vi "argosclient.vi"() -> ()   [LabVIEW 2014]
panel:
  out "locking":string
  in  "stop":bool
  out "bscale":dbl format="%#_9g"
  in  "set locking":bool
  in  "wnum setpoint":dbl=2284.249 format="%#_13g"
  in  "bscale":dbl=1.0 min=0.0001 max=1.0 step=0.0001 format="%#_13g"
  in  "locking":enum16{"off", "reg a", "reg b"}(ring)
  out "wnum measured":dbl format="%#_9g"
  in  "set bscale":bool
  in  "set wnum":bool
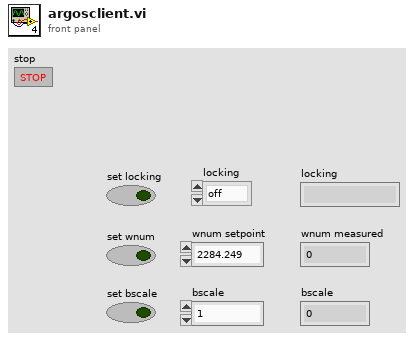
[diagram p1: front panel]
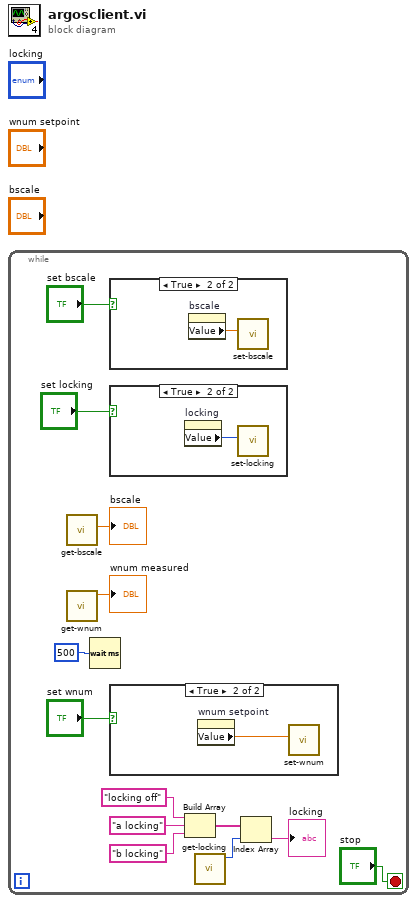
[diagram p0: block diagram]
diagram:
  n1 = while {
    stop <- "stop" stop-if-true
    n2 = call "get-bscale.vi"() -> ("bscale"=→"bscale":dbl)  [unwired: 10 in, 1 out]
    n3 = call "get-wnum.vi"() -> ("wnum"=→"wnum measured":dbl)  [unwired: 10 in, 1 out]
    n4 = Wait (ms)(milliseconds to wait=u32 500) -> ()  [unwired: 1 out]
    n5 = case shown="True" "set bscale" {
      frame False {
      }
      frame True {
        n6 = property on="bscale" class="DigNum (strict)"() -> ("Value"=w15:dbl)  [unwired: 2 in, 2 out]
        n7 = call "set-bscale.vi"("bscale"=w15) -> ()  [unwired: 10 in, 1 out]
      }
    }
    n8 = case shown="True" "set locking" {
      frame False {
      }
      frame True {
        n9 = property on="locking" class="Enum (strict)"() -> ("Value"=w14:enum16{"off", "reg a", "reg b"})  [unwired: 2 in, 2 out]
        n10 = call "set-locking.vi"("locking"=w14) -> ()  [unwired: 10 in, 1 out]
      }
    }
    n11 = case shown="True" "set wnum" {
      frame False {
      }
      frame True {
        n12 = property on="wnum setpoint" class="DigNum (strict)"() -> ("Value"=w16:dbl)  [unwired: 2 in, 2 out]
        n13 = call "set-wnum.vi"("wnum"=w16) -> ()  [unwired: 10 in, 1 out]
      }
    }
    n14 = Build Array("locking off", "a locking", "b locking") -> (w2:string[])
    n15 = call "get-locking.vi"() -> ("locking"=w3:u8)  [unwired: 10 in, 1 out]
    n16 = Index Array(array=w2, index=w3) -> (element=→"locking":string)
  }
